vi "AiToFIFO.vi"(1 "FIFO":refnum<k21>="AI-DRAM FIFO 0", 2 "FPGA I/O 1":refnum<k21>="IO Module\\AI A1", 3 "FPGA I/O 0":refnum<k21>="IO Module\\AI A1") -> (0 "Overflow":bool)   [LabVIEW 2014]
doc: "Store two AI channels in a FIFO.\n\nAI channels are sampled at 50MHz, DRAM memory reads at 100MHz."
uses:
  <vilib>/rvi/eio/common/nirviEmuTemplateMethod_errors.vi
  <vilib>/rvi/DataTransferAndStorage/Container/Common/niFpgaContainerExecOnDevCompGetState.vi
  <vilib>/rvi/Emulation/niFpgaEmulationIsFPGAContextNoSignature.vi
  <vilib>/rvi/Emulation/niFpgaSctlEmulationGetInTimedLoop.vi
  <vilib>/rvi/errors/niFpgaSetErrorForExecOnDevCompSimple.vi
  <vilib>/rvi/eio/common/nirviEmuReportErrorAndStop.vi
  <vilib>/rvi/DataTransferAndStorage/Container/Common/niFpgaContainerGetUniqueNameForEmu.vi
  <vilib>/rvi/FIFO/Fifo_Resource/nirvififoEmulationSetSize.vi
  <vilib>/rvi/FIFO/Fifo_Resource/nirviFifoEmulationQueueMgr.vi
  <instcachedir>/0/nirviFifoEmulationQueueMgr_E5CAEC123FF24DC58D834DCA3CDAA9B5.lvgen/nirviFifoEmulationQueueMgr_E5CAEC123FF24DC58D834DCA3CDAA9B5_002.vi
  <vilib>/rvi/FIFO/Fifo_Resource/nirvififoEmulationDetermineInputValidOut.vi
  <vilib>/rvi/FIFO/Fifo_Resource/nirvififoEmulationCreateLock.vi
  <vilib>/rvi/Emulation/niFpgaProcessEmulError.vi
  <vilib>/rvi/FIFO/Fifo_Resource/nirvififoEmulationObtainLock.vi
  <vilib>/rvi/FIFO/Fifo_Resource/nirvififoEmulationReleaseLock.vi
  <vilib>/rvi/occurrence/nirviWaitOnOccurrenceBase.vi
  <vilib>/rvi/errors/nirviReportUnexpectedCaseInternalError.vi
  <vilib>/rvi/errors/nirviReportUnexpectedCaseInternalError (U32).vi
  <vilib>/Utility/error.llb/Clear Errors.vi
  <vilib>/rvi/interface/RandomDataEmulation/niFpgaRandomDataHandleErrors.vi
  <vilib>/eio/EIONode/EIONode.xnode
  <vilib>/rvi/DataTransferAndStorage/Container/XNode/niFpgaContainer.xnode
  <vilib>/rvi/FIFO/Fifo_Resource/niFpgaFifoEmulationRefIn.vi
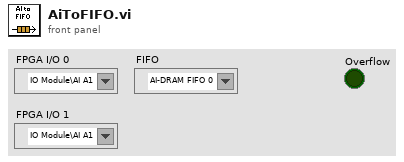
[diagram p1: front panel]
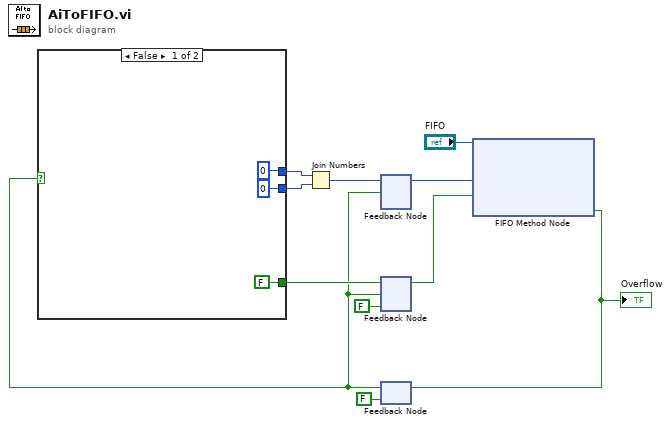
[diagram p0: block diagram]
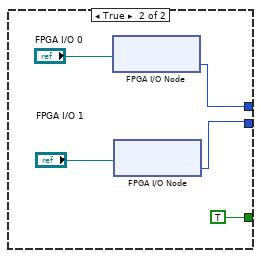
[diagram p2: hidden frame]
diagram:
  n1 = feedback #1() -> (w6:u32)  [unwired: 1 in]
  n2 = feedback #2(FALSE) -> (w4:bool)
  n3 = feedback #3(FALSE ("Ready for Input")) -> (w2:bool)
  n4 = case shown="False" w2 {
    tunnel: [i16 0 ("I/O Item") w17] -> w10
    tunnel: [i16 0 ("I/O Item") w16] -> w9
    tunnel: [FALSE TRUE] -> w5
    frame False {
    }
    frame True {
      n5 = xnode "FPGA I/O Node"("FPGA I/O In"="FPGA I/O 0") -> ("I/O Item"=w16:i16)  [unwired: 1 out]
      n6 = xnode "FPGA I/O Node"("FPGA I/O In"="FPGA I/O 1") -> ("I/O Item"=w17:i16)  [unwired: 1 out]
    }
  }
  n7 = Join Numbers(hi=w9, lo=w10) -> ((hi.lo)=w7:u32)
  n8 = feedback-in #1(w7, w2) -> ()
  n9 = feedback-in #2(w5, w2) -> ()
  n10 = xnode ("FIFO Method Node")("Element"=w6, "Input Valid"=w4, "FIFO In"="FIFO") -> ("Ready for Input"=w8:bool)  [unwired: 1 in, 2 out]
  "Overflow" <- w8
  n11 = feedback-in #3(w8) -> ()
